vi "REV_Velocity PID Single Motor with streams.vi"() -> ()   [LabVIEW 2020]
doc: "Use this example VI to tune a single SPARK MAX motor controller.\n\nThis example should be placed in 'Periodic Tasks.vi' and used during testing only. Make sure the motor controller has been opened and configured before this is called."
uses:
  <vilib>/Rock Robotics/WPI/ThirdParty/REV Robotics/REVLib/Typedef/Spark MAX Control Type.ctl
panel:
  in  "Setpoint":dbl(slide) scale=-5700.0..5700.0
  out "PID Chart":T1(graph)
  in  "PID Constants":T2={"P Gain"=0.0, "I Gain"=0.0, "D Gain"=0.0, "F Gain"=0.0, "I Zone"=0.0, "Min Output"=-1.0, "Max Output"=1.0} {"Max Output" min=-1.0 max=1.0 step=0.01; "Min Output" min=-1.0 max=1.0 step=0.01; "I Zone" step=0.01; "F Gain" step=0.01; "D Gain" step=0.01; "I Gain" step=0.01; "P Gain" min=0.0 step=0.01}
  # "Click here to set max"
  # "Click here to set min"
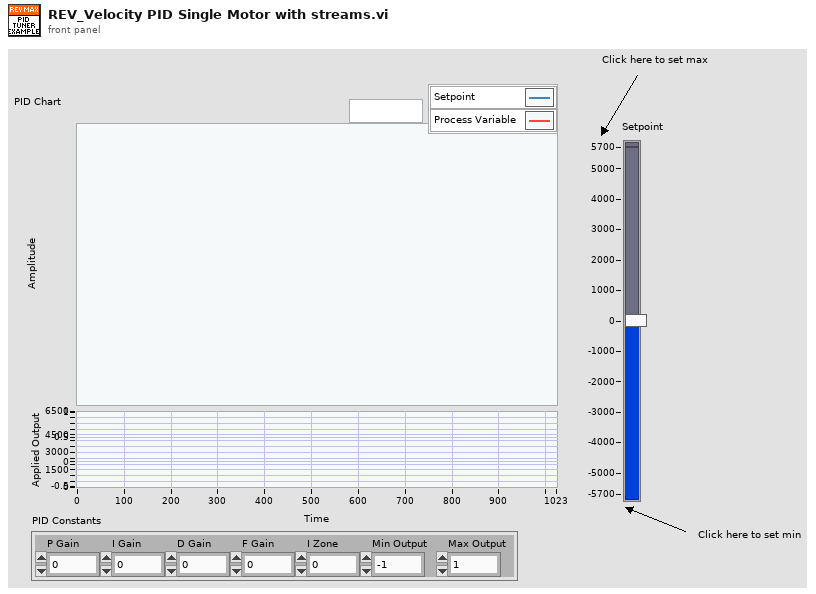
[diagram p1: front panel]
types:
  T1 = cluster{"Sensor Velocity":dbl, "Setpoint":dbl, "Applied Output":dbl}
  T2 = cluster{"P Gain":dbl, "I Gain":dbl, "D Gain":dbl, "F Gain":dbl, "I Zone":dbl, "Min Output":dbl, "Max Output":dbl}
  T3 = typedef "WPI_MotorControlDeviceRef.ctl" = cluster{"DeviceStatus":errorcluster, "Type":T4, "PWM":cluster{"PWM Channel":T5, "DeadBand":T6}, "CAN":cluster{"Device Number":u8, "SetOutput VI Ref":variant, "GetOutput VI Ref":variant, "Enable VI Ref":variant, "Disable VI Ref":variant, "Data":variant}, "Invert":bool, "DIO PWM":cluster{"PWM \"Enable\" Channel":T5, "DIOChannel":T7, "PWM Rate":dbl}}
  T4 = typedef "WPI_MotorControlType.ctl" = enum16{"PWM", "CAN", "DIO PWM"}
  T5 = typedef "FPGA_DIOPWMChannel.ctl" = enum8{"PWM 0", "PWM 1", "PWM 2", "PWM 3", "PWM 4", "PWM 5", "PWM 6", "PWM 7", "PWM 8", "PWM 9", "PWM MXP 0", "PWM MXP 1", "PWM MXP 2", "PWM MXP 3", "PWM MXP 4", "PWM MXP 5", "PWM MXP 6", "PWM MXP 7", "PWM MXP 8", "PWM MXP 9", "Invalid"}
  T6 = typedef "WPI_PWMDeadband.ctl" = cluster{"Name":string, "maxPositivePwm":i32, "minPositivePwm":i32, "centerPwm":i32, "maxNegativePwm":i32, "minNegativePwm":i32, "angularRange":u16}
  T7 = typedef "FPGA_DIOChannel.ctl" = enum8{"DIO 0", "DIO 1", "DIO 2", "DIO 3", "DIO 4", "DIO 5", "DIO 6", "DIO 7", "DIO 8", "DIO 9", "DIO MXP 0", "DIO MXP 1", "DIO MXP 2", "DIO MXP 3", "DIO MXP 4", "DIO MXP 5", "DIO MXP 6", "DIO MXP 7", "DIO MXP 8", "DIO MXP 9", "DIO MXP 10", "DIO MXP 11", "DIO MXP 12", "DIO MXP 13", "DIO MXP 14", "DIO MXP 15", "SPI Port CS1", "SPI Port CS2", "SPI Port CS3", "SPI Port MISO", "SPI Port MOSI", "Invalid"}
  T8 = typedef "Spark MAX Control Type.ctl" = enum16{"Percent VBus", "Voltage", "Velocity", "Position", "Smart Motion", "Current", "Smart Velocity"}
  T9 = cluster{"P Gain":bool, "I Gain":bool, "D Gain":bool, "F Gain":bool, "I Zone":bool, "Min Output":bool, "Max Output":bool}
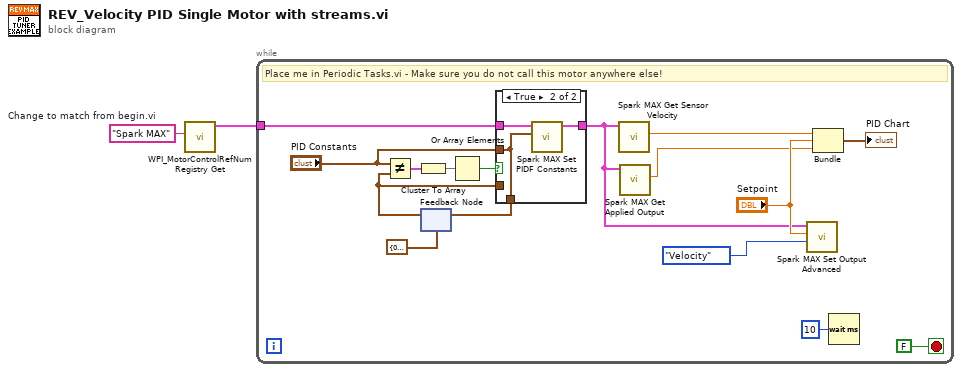
[diagram p0: block diagram]
diagram:
  w2 = "Spark MAX"  # Change to match from begin.vi
  n1 = call <vilib>:"WPI_MotorControlRefNum Registry Get.vi"("refnum name"=w2) -> ("MotorControlDevRef"=w1:T3)  [unwired: 9 in, 1 out]
  n2 = while {
    tunnel: w1 -> [w8]
    stop <- FALSE stop-if-true
    # "Place me in Periodic Tasks.vi - Make sure you do not call this motor anywhere else!"
    n3 = feedback #1(T2 {"P Gain"=0.0, "I Gain"=0.0, "D Gain"=0.0, "F Gain"=0.0, "I Zone"=0.0, "Min Output"=0.0, "Max Output"=0.0} ("PID Constants")) -> (w15:T2)
    n4 = Not Equal?(x="PID Constants", y=w15) -> (x != y?=w9:T9)
    n5 = Cluster To Array(cluster=w9) -> (array=w10:bool[])
    n6 = Or Array Elements(Boolean array=w10) -> (logical OR=w12:bool)
    n7 = case shown="True" w12 {
      tunnel: w8 -> [w19 w23]
      tunnel: "PID Constants" -> [_ w21]
      tunnel: [w20 w21] -> w14
      tunnel: w15 -> [w20 _]
      tunnel: [w19 w22] -> w3
      frame False {
      }
      frame True {
        n8 = call <vilib>:"Spark MAX Set PIDF Constants.vi"("PID Constants"=w21, "MotorControlDeviceRef"=w23) -> ("MotorControlDeviceRef"=w22:T3)  [unwired: 8 in, 1 out]
      }
    }
    n9 = feedback-in #1(w14) -> ()
    n10 = call <vilib>:"Spark MAX Get Sensor Velocity.vi"("MotorControlDevRef in"=w3) -> ("Sensor Velocity"=w5:dbl)  [unwired: 7 in, 3 out]
    n11 = call <vilib>:"Spark MAX Get Applied Output.vi"("MotorControlDevRef in"=w3) -> ("Applied Output"=w4:dbl)  [unwired: 7 in, 3 out]
    n12 = call <vilib>:"Spark MAX Set Output Advanced.vi"("Control Mode"=Spark_MAX_Control_Type."Velocity", "Setpoint"="Setpoint", "MotorControlDevRef"=w3) -> ()  [unwired: 7 in, 2 out]
    n13 = Bundle("Sensor Velocity"=w5, "Setpoint"="Setpoint", "Applied Output"=w4) -> (→"PID Chart":T1)  [unwired: 1 in]
    n14 = Wait (ms)(milliseconds to wait=u32 10) -> ()  [unwired: 1 out]
  }
